vi "calculate  checksum.vi"(11 "front command":u8[](array[numeric]) format="%02x") -> (0 "DATA":u8[](array[numeric]) format="%02x", 3 "校验位":u8 format="%02x")   [LabVIEW 2013]
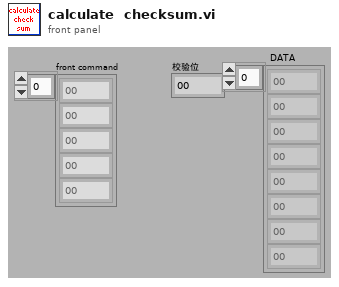
[diagram p1: front panel]
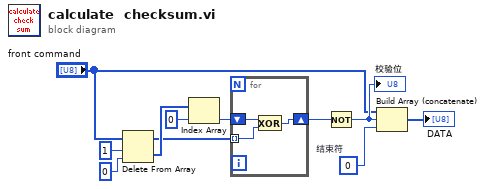
[diagram p0: block diagram]
diagram:
  w3 = u8 0  # 结束符
  n1 = Delete From Array(array="front command", length=1 ("长度"), index=0 ("索引")) -> (deleted portion=w9:u8[], array with subset deleted=w5:u8[])
  n2 = Index Array(array=w9, index=0 ("索引")) -> (element=w6:u8)
  n3 = for {
    tunnel: w5 -> [w14] mode=indexing
    shift-right: [w13] -> w11
    shift-left: w6 -> [w12]
    n4 = Exclusive Or(1:w14, 2:w12) -> (0:w13:u8)
  }
  n5 = Not(x=w11) -> (.not. x?=w4:u8)
  "校验位" <- w4
  n6 = Build Array (concatenate)("front command", w4, w3) -> (→"DATA":u8[])
